vi "sccx.vi"(0 "IP adress":string="192.109.209.229", 1 "stop":bool, 2 "Channel":u8(ring) items=["1", "2", "3", "4", "5", "6", "7", "8", "9", "10", "11", "12", "13", "14", "15", "16"], 4 "Exit":bool, 5 "Start":bool, 6 "Draw":enum16{"Ewe(t)", "Ece(t)", "I(t)", "Q(t)"}(ring)) -> (7 "XY Graph":cluster{"Data 101":sgl[], "Data 101":sgl[]}(graph), 8 "Number of points":i32=1992)   [LabVIEW 2012]
doc: "Chrono-Amperometry (CA) is a controlled-potential technique. The current response is measured to an applied potential step.\nIn general, in this VI, the first thing to do is to start by establishing the connection with the instrument defined by its IP adress, then load the firmware in the channel selected, get the information on the plugged channels, load protocol on a channel, start/stop the protocol, retreive data and draw the graph."
uses:
  base_xml.llb/Type Descriptor Enumeration__ogtk.ctl
panel:
  in  "SCCX Parameters":T1={"I_Range"=11, "E_Range"=0, "Bandwidth"=3, "par_E0"=1.0, "par_A"=0.0, "par_B"=0.1, "par_QRP_select"=1, "par_E_duration"=0.01, "par_E_dt_rec"=0.0001, "par_I0_duration"=0.01, "par_I0_dt_rec"=0.0001, "par_NC"=9, "par_RC"=1, "par_Q_limit_val"=5e-05, "par_Q_limit_cfg"=0, "par_QRP_time"=0.005, "ce"=0, "em"=0} {"par_Q_limit_cfg" items=["Disable"=0, "Enable if <"=129, "Enable if >"=133]; "par_QRP_select" items=["Ewe", "Ece"]; "E_Range" items=["±2.5V", "±5V", "±10V", "Auto"]; "Bandwidth" items=["1"=1, "2"=2, "3"=3, "4"=4, "5"=5, "6"=6, "7"=7, "8"=8, "9"=9]; "I_Range" items=["1pA", "1nA", "10nA", "100nA", "1µA", "10µA", "100µA", "1mA", "10mA", "100mA", "1A", "Booster", "Auto"]}
  out "Exit 2":bool=TRUE
  out "Data 101":sgl[][](array[numeric]) format="%.2f"
  # "Instructions:\nBefore running the VI you must type a valid IP adress that corresponds to the instrument.Then press the Run button to execute this VI.\nWhile this VI is running, choose the available channel, enter the CA parameters or keep the default values, then press the start button to begin the experience.\nChoose the waveform to draw (Ewe(t) or I(t)). You can stop the measure if you press the stop button and exit the execution if you press the exit button."
  # "V"
  # "Next En+1 = En - B * (A - QRP)"
  # "s"
  # "s"
  # "Switch to  I = 0"
  # "s"
  # "s"
  # "s"
  # "C"
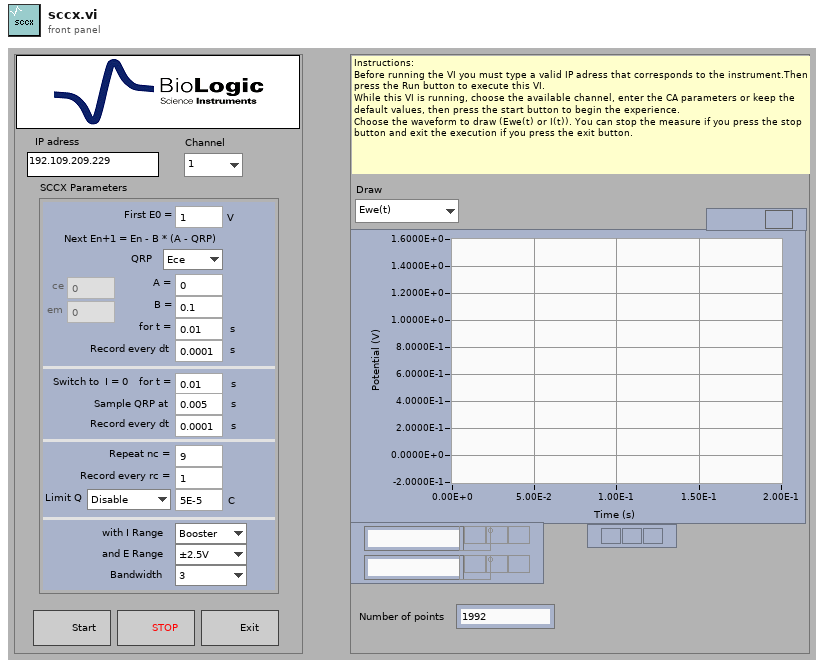
[diagram p1: front panel]
types:
  T1 = cluster{"I_Range":u16, "E_Range":u16, "Bandwidth":u16, "par_E0":sgl, "par_A":sgl, "par_B":sgl, "par_QRP_select":u16, "par_E_duration":sgl, "par_E_dt_rec":sgl, "par_I0_duration":sgl, "par_I0_dt_rec":sgl, "par_NC":i32, "par_RC":i32, "par_Q_limit_val":sgl, "par_Q_limit_cfg":u16, "par_QRP_time":sgl, "ce":i32, "em":i32}
  T2 = typedef "Type Descriptor Enumeration__ogtk.ctl" = enum8{"<Null>", "I8", "I16", "I32", "I64", "U8", "U16", "U32", "U64", "SGL", "DBL", "EXT", "CSG", "CDB", "CXT", "0x0F", "0x10", "0x11", "0x12", "0x13", "0x14", "Enum U8", "Enum U16", "Enum U32", "Enum U64", "SGL PQ", "DBL PQ", "EXT PQ", "CSG PQ", "CDB PQ", "CXT PQ", "0x1F", "0x20", "Boolean", "0x22", "0x23", "0x24", "0x25", "0x26", "0x27", "0x28", "0x29", "0x2A", "0x2B", "0x2C", "0x2D", "0x2E", "0x2F", "String", "0x31", "Path", "Pict", "0x34", "0x35", "0x36", "DAQ", "0x38", "0x39", "0x3A", "0x3B", "0x3C", "0x3D", "0x3E", "0x3F", "Array", "0x41", "0x42", "0x43", "0x44", "0x45", "0x46", "0x47", "0x48", "0x49", "0x4A", "0x4B", "0x4C", "0x4D", "0x4E", "0x4F", "Cluster", "0x51", "0x52", "Variant", "Waveform", "0x55", "0x56", "0x57", "0x58", "0x59", "0x5A", "0x5B", "0x5C", "0x5D", "0x5E", "0x5F", "0x60", "0x61", "0x62", "0x63", "0x64", "0x65", "0x66", "0x67", "0x68", "0x69", "0x6A", "0x6B", "0x6C", "0x6D", "0x6E", "0x6F", "Refnum"}
  T3 = cluster{"Data Type":T2, "Format String":string}[]
  T4 = cluster{"Channel":i32, "BoardVersion":i32, "BoardSerialCode":i32, "FirmwareCode":i32, "FirmwareVersion":i32, "XilinxVersion":i32, "AmpCode":i32, "NbAmp":i32, "LcBoard":i32, "Zboard":i32, "MuxBoard":i32, "GPRAboard":i32, "MemSize":i32, "MemFilled":i32, "state":i32, "MaxIRange":i32, "MinIRange":i32, "MaxBandwidth":i32, "NbOfTechniques":i32}
  T5 = cluster{"Label":string, "type":i32, "valeur":u32, "index":i32}[]
  T6 = cluster{"IRQskipped":i32, "NbRaws":i32, "NbCols":i32, "Technique Index":i32, "TechniqueID":i32, "PrcessIndex":i32, "loop":i32, "StartTime":dbl, "MuxPad":i32}
  T7 = cluster{"State":i32, "MemFilled":i32, "TimeBase":sgl, " Ewe":sgl, " EweRangeMin":sgl, " EweRangeMax":sgl, "Ece":sgl, "EceRangeMin":sgl, "EceRangeMax":sgl, "Eoverflow":i32, "I":sgl, "IRange":i32, "Ioverflow":i32, "ElapsedTime":sgl, "Freq":sgl, "Rcomp":sgl, "Saturation":sgl, "OptErr":i32, "OptPos":i32}
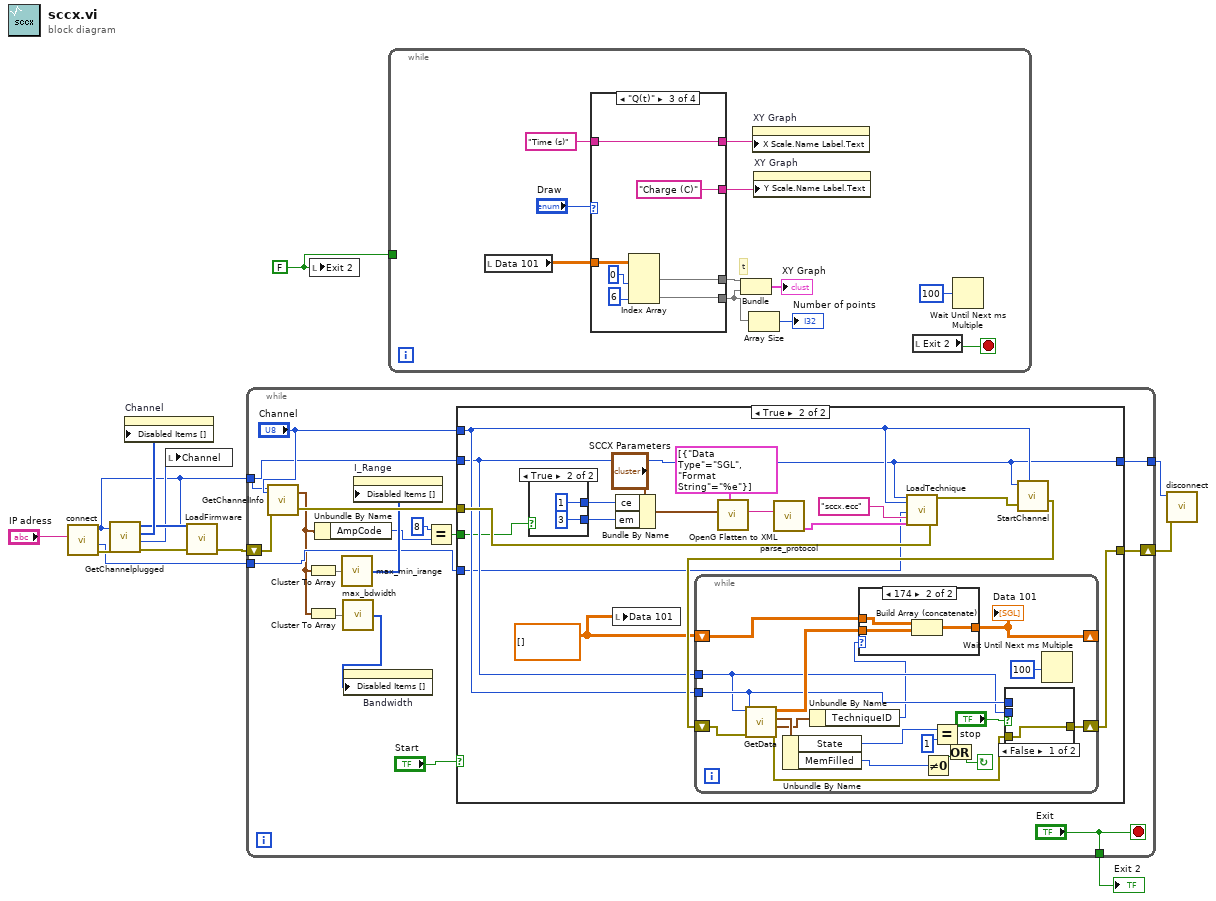
[diagram p0: block diagram]
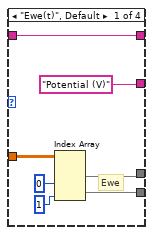
[diagram p2: hidden frame]
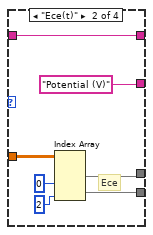
[diagram p3: hidden frame]
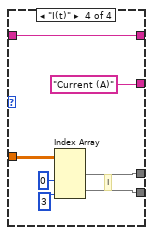
[diagram p4: hidden frame]
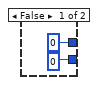
[diagram p6: hidden frame]
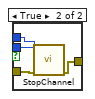
[diagram p7: hidden frame]
diagram:
  w12 = FALSE ("Exit 2")
  n1 = call "connect.vi"("IP"="IP adress") -> ("error out"=w10:errorcluster, "Device Code"=w1:i32, "ID"=w3:i32)  [unwired: 7 in, 1 out]
  n2 = call "GetChannelplugged.vi"("error in (no error)"=w10, "ID"=w3) -> ("error out"=w7:errorcluster, "First channel"=w5:i32, "Disabled channels"=w9:i32[], "Plugged channels"=w8:i32[])  [unwired: 6 in]
  n3 = property on="Channel" class="Ring (strict)"("Disabled Items []"=w9) -> ()  [unwired: 2 in, 2 out]
  n4 = local write "Channel"(w5) -> ()
  n5 = call "LoadFirmware.vi"("error in (no error)"=w7, "Channels"=w8, "ID"=w3) -> ("error out"=w4:errorcluster)  [unwired: 7 in, 1 out]
  n6 = while {
    shift-right: [w29] -> w11
    shift-left: w4 -> [w26]
    tunnel: ["Exit"] -> w13
    tunnel: w3 -> [w22]
    tunnel: [w21] -> w2
    tunnel: w1 -> [w18]
    stop <- "Exit" stop-if-true
    n7 = call "GetChannelInfo.vi"("error in (no error)"=w26, "Channel"="Channel", "ID"=w22) -> ("error out"=w25:errorcluster, "Channel information"=w17:T4)  [unwired: 7 in]
    n8 = Cluster To Array(cluster=w17) -> (array=w24:i32[])
    n9 = Cluster To Array(cluster=w17) -> (array=w23:i32[])
    n10 = Unbundle By Name(w17) -> ("AmpCode"=w15:i32)
    n11 = call "max_min_irange.vi"("resources"=w24) -> ("disabled ranges"=w19:i32[])
    n12 = call "max_bdwidth.vi"("resources"=w23) -> ("disabled ranges"=w20:i32[])
    n13 = property on="Bandwidth" class="Ring (strict)"("Disabled Items []"=w20) -> ()  [unwired: 2 in, 2 out]
    n14 = property on="I_Range" class="Ring (strict)"("Disabled Items []"=w19) -> ()  [unwired: 2 in, 2 out]
    n15 = Equal?(x=8, y=w15) -> (x = y?=w14:bool)
    n16 = case shown="True" "Start" {
      tunnel: "Channel" -> [_ w43]
      tunnel: [w32 w46] -> w29
      tunnel: w25 -> [w32 w45]
      tunnel: w22 -> [w31 w39]
      tunnel: [w31 w39] -> w21
      tunnel: w18 -> [_ w38]
      tunnel: w14 -> [_ w37]
      frame False {
      }
      frame True {
        w44 = sgl[][] []
        n17 = case shown="True" w37 {
          tunnel: [0 ("ce") 1 ("ce")] -> w34
          tunnel: [0 ("ce") 3 ("ce")] -> w33
          frame False {
          }
          frame True {
          }
        }
        n18 = local write "Data 101"(w44) -> ()
        n19 = Bundle By Name(cluster="SCCX Parameters", "ce"=w34, "em"=w33) -> (w35:T1)
        n20 = call "OpenG Flatten to XML.vi"("Type Formats (default)"=T3 [{"Data Type"=enum."SGL", "Format String"="%e"}] ("Type Formats"), "LabVIEW Data"=w35) -> ("XML String"=w42:string)  [unwired: 8 in, 1 out]
        n21 = call "parse_protocol.vi"("XML String In"=w42) -> ("Params Values"=w41:T5)  [unwired: 8 in]
        n22 = call "LoadTechnique.vi"("ID"=w39, "Selected Channel"=w43, "Device Code"=w38, "FName"="sccx.ecc", "Protocol Parameters"=w41, "error in (no error)"=w45) -> ("error out"=w48:errorcluster)  [unwired: 13 in]
        n23 = call "StartChannel.vi"("error in (no error)"=w48, "Channel"=w43, "ID"=w39) -> ("error out"=w47:errorcluster)  [unwired: 8 in]
        n24 = while {
          shift-right: [w66] -> w46
          shift-left: w47 -> [w69]
          shift-right: [w63] -> _
          shift-left: w44 -> [w64]
          tunnel: w43 -> [w60]
          tunnel: w39 -> [w59]
          stop <- w67 continue-if-true
          n25 = call "GetData.vi"("error in (no error)"=w69, "Channel"=w60, "ID"=w59) -> ("error out"=w62:errorcluster, "Data information"=w55:T6, "Current values"=w58:T7, "Data"=w65:dbl[][])  [unwired: 5 in]
          n26 = Unbundle By Name(w58) -> ("State"=w57:i32, "MemFilled"=w56:i32)
          n27 = Unbundle By Name(w55) -> ("TechniqueID"=w54:i32)
          n28 = case shown="174" w54 {
            tunnel: w65 -> [_ w81]
            tunnel: w64 -> [w78 w80]
            tunnel: [w78 w79] -> w63
            frame 0, Default {
            }
            frame 174 {
              n29 = Build Array (concatenate)(w80, w81) -> (w79:dbl[][])
            }
          }
          "Data 101" <- w63
          n30 = Not Equal To 0?(x=w56) -> (x != 0?=w70:bool)
          n31 = Equal?(x=w57, y=1) -> (x = y?=w71:bool)
          n32 = Or(x=w71, y=w70) -> (x .or. y?=w67:bool)
          n33 = case shown="False" "stop" {
            tunnel: [w73 w77] -> w66
            tunnel: w62 -> [w73 w76]
            tunnel: w60 -> [_ w75]
            tunnel: w59 -> [_ w74]
            frame False {
            }
            frame True {
              n34 = call "StopChannel.vi"("error in (no error)"=w76, "Channel"=w75, "ID"=w74) -> ("error out"=w77:errorcluster)  [unwired: 8 in]
            }
          }
          n35 = Wait Until Next ms Multiple(millisecond multiple=u32 100) -> ()  [unwired: 1 out]
        }
      }
    }
  }
  "Exit 2" <- w13
  n36 = local write "Exit 2"(w12) -> ()
  n37 = while {
    tunnel: w12 -> [_]
    stop <- w91 stop-if-true
    # "t"
    n38 = local read "Data 101"() -> (w86:sgl[][])
    n39 = case shown="\"Q(t)\"" "Draw" {
      tunnel: ["Potential (V)" ("Y Scale.Name Label.Text") "Potential (V)" ("Y Scale.Name Label.Text") "Charge (C)" ("Y Scale.Name Label.Text") "Current (A)" ("Y Scale.Name Label.Text")] -> w89
      tunnel: [w99 w106 w113 w120] -> w88
      tunnel: "Time (s)" ("Y Scale.Name Label.Text") -> [w99 w106 w113 w120]
      tunnel: w86 -> [w96 w103 w111 w117]
      tunnel: [w94 w101 w108 w115] -> w84
      tunnel: [w93 w100 w107 w114] -> w83
      frame "Ewe(t)", Default {
        # "Ewe"
        n40 = Index Array(array=w96, index (col) #1=0 ("Index"), index (col) #2=1 ("Index")) -> (element #1=w94:sgl[], element #2=w93:sgl[])  [unwired: 2 in]
      }
      frame "Ece(t)" {
        # "Ece"
        n41 = Index Array(array=w103, index (col) #1=0 ("Index"), index (col) #2=2 ("Index")) -> (element #1=w101:sgl[], element #2=w100:sgl[])  [unwired: 2 in]
      }
      frame "Q(t)" {
        n42 = Index Array(array=w111, index (col) #1=0 ("Index"), index (col) #2=6 ("indice désactivé (col)")) -> (element #1=w108:sgl[], element #2=w107:sgl[])  [unwired: 2 in]
      }
      frame "I(t)" {
        # "I"
        n43 = Index Array(array=w117, index (col) #1=0 ("Index"), index (col) #2=3 ("indice désactivé (col)")) -> (element #1=w115:sgl[], element #2=w114:sgl[])  [unwired: 2 in]
      }
    }
    n44 = Bundle("Data 101"=w84, "Data 101"=w83) -> (→"XY Graph":cluster{"Data 101":sgl[], "Data 101":sgl[]})  [unwired: 1 in]
    n45 = Array Size(array=w83) -> (size(s)=→"Number of points":i32)
    n46 = property on="XY Graph" class="XYGraph (strict)"("X Scale.Name Label.Text"=w88) -> ()  [unwired: 2 in, 2 out]
    n47 = property on="XY Graph" class="XYGraph (strict)"("Y Scale.Name Label.Text"=w89) -> ()  [unwired: 2 in, 2 out]
    n48 = local read "Exit 2"() -> (w91:bool)
    n49 = Wait Until Next ms Multiple(millisecond multiple=u32 100) -> ()  [unwired: 1 out]
  }
  n50 = call "disconnect.vi"("error in (no error)"=w11, "ID"=w2) -> ()  [unwired: 9 in, 1 out]
